vi "xps_panel_DO_generate_pvt_trajectory.vi"(7 "Dither Cycles":u32=3, 8 "error in (no error)":errorcluster, 9 "custom?":bool=TRUE, 10 "Custom Dither Trajectory":T1 {"Dither Period (s)" min=0.0; "PVT Ampl (nm)" min=0.0}, 11 "newport_xps_panel in":refnum<class "newport_xps_panel.lvclass">) -> (0 "error out":errorcluster, 3 "newport_xps_panel out":refnum<class "newport_xps_panel.lvclass">)   [LabVIEW 2015, in "newport_xps_panel.lvclass"]
uses:
  newport_xps_panel.lvclass
  newport_xps/dither_trajectory_settings.ctl
  newport_xps/dither_trajectory_types.ctl
  newport_xps/newport_xps.lvclass
  UI/panel_class/panel.lvclass
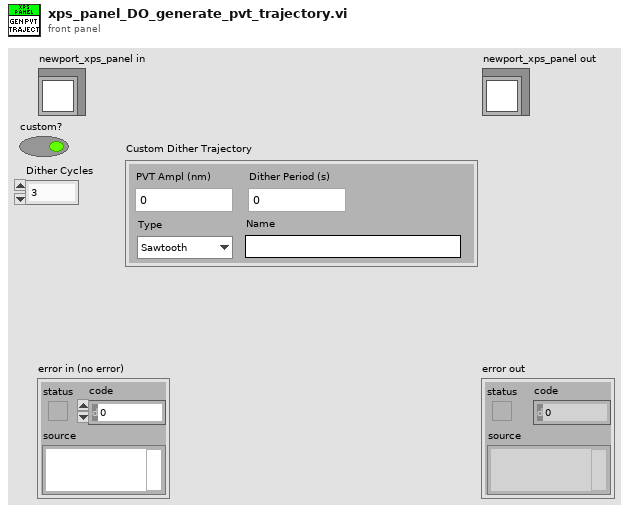
[diagram p1: front panel]
types:
  T1 = typedef "dither_trajectory_settings.ctl" = cluster{"PVT Ampl (nm)":dbl, "Dither Period (s)":dbl, "Type":T2, "Name":string}
  T2 = typedef "dither_trajectory_types.ctl" = enum16{"Sawtooth"}
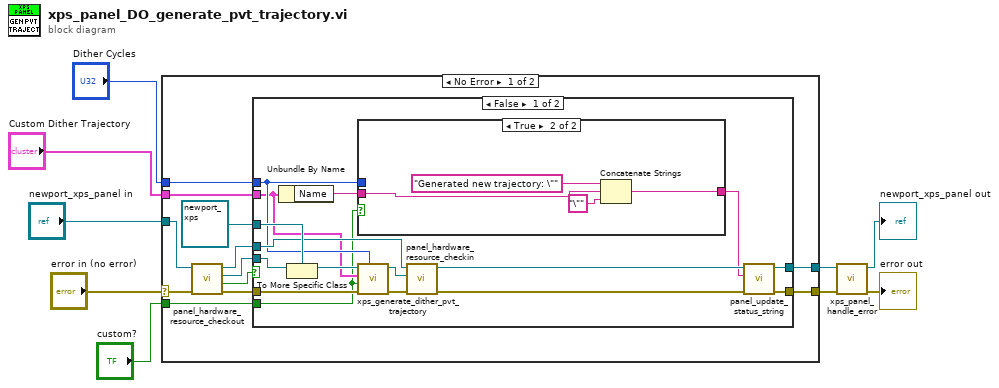
[diagram p0: block diagram]
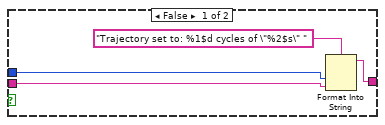
[diagram p2: hidden frame]
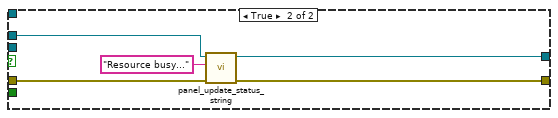
[diagram p3: hidden frame]
diagram:
  n1 = case shown="No Error" "error in (no error)" {
    selector: "error in (no error)" -> [w21 w52]
    tunnel: [w15 w52] -> w7
    tunnel: [w14 w51] -> w5
    tunnel: "newport_xps_panel in" -> [w20 w51]
    tunnel: "Custom Dither Trajectory" -> [w12 _]
    tunnel: "custom?" -> [w11 _]
    tunnel: "Dither Cycles" -> [w10 _]
    frame No Error {
      n2 = call "panel_hardware_resource_checkout.vi"("error in (no error)"=w21, "panel in"=w20) -> ("error out"=w16:errorcluster, "timed out?"=w19:bool, "hardware.lvclass"=w17:refnum<class "hardware.lvclass">, "panel out"=w18:refnum<class "newport_xps_panel.lvclass">)  [unwired: 6 in]
      n3 = case shown="False" w19 {
        tunnel: w18 -> [w31 w47]
        tunnel: w17 -> [w37 _]
        tunnel: w16 -> [w27 w50]
        tunnel: [w33 w49] -> w15
        tunnel: [w32 w46] -> w14
        tunnel: refnum<class "newport_xps.lvclass"> refnum ("newport_xps in") -> [w36 _]
        tunnel: w12 -> [w25 _]
        tunnel: w11 -> [w22 _]
        tunnel: w10 -> [w26 _]
        frame False {
          n4 = Unbundle By Name(w25) -> ("Name"=w24:string)
          n5 = To More Specific Class(target class=w36, reference=w37) -> (specific class reference=w30:refnum<class "newport_xps.lvclass">)  [unwired: 1 in, 1 out]
          n6 = case shown="True" w22 {
            tunnel: w26 -> [w40 _]
            tunnel: w24 -> [w39 w44]
            tunnel: [w38 w42] -> w23
            frame False {
              n7 = Format Into String(format string="Trajectory set to: %1$d cycles of \"%2$s\" " ("string"), w40, w39) -> (resulting string=w38:string)  [unwired: 2 in, 1 out]
            }
            frame True {
              n8 = Concatenate Strings("Generated new trajectory: \"" ("string"), w44, "\"" ("string")) -> (w42:string)
            }
          }
          n9 = call "xps_generate_dither_pvt_trajectory.vi"("Dither Cycles"=w26, "error in (no error)"=w27, "custom?"=w22, "Custom Dither Trajectory"=w25, "newport_xps in"=w30) -> ("error out"=w28:errorcluster, "newport_xps out"=w29:refnum<class "newport_xps.lvclass">)  [unwired: 5 in]
          n10 = call "panel_hardware_resource_checkin.vi"("error in (no error)"=w28, "hardware.lvclass"=w29, "panel in"=w31) -> ("error out"=w35:errorcluster, "panel out"=w34:refnum<class "newport_xps_panel.lvclass">)  [unwired: 7 in]
          n11 = call-dynamic "panel_update_status_string.vi"("error in (no error)"=w35, "String"=w23, "newport_xps_panel in"=w34) -> ("error out"=w33:errorcluster, "newport_xps_panel out"=w32:refnum<class "newport_xps_panel.lvclass">)  [unwired: 7 in]
        }
        frame True {
          n12 = call-dynamic "panel_update_status_string.vi"("error in (no error)"=w50, "String"="Resource busy...", "newport_xps_panel in"=w47) -> ("error out"=w49:errorcluster, "newport_xps_panel out"=w46:refnum<class "newport_xps_panel.lvclass">)  [unwired: 7 in]
        }
      }
    }
    frame Error {
    }
  }
  n13 = call "xps_panel_handle_error.vi"("error in (no error)"=w7, "newport_xps_panel in"=w5) -> ("error out"=→"error out":errorcluster, "newport_xps_panel out"=→"newport_xps_panel out":refnum<class "newport_xps_panel.lvclass">)  [unwired: 8 in]
